vi "Close_Refs.vi"(8 "Error In":errorcluster caption="Entrée d'erreur", 11 "Donnees_Globales_IN":T1) -> (0 "Error Out":errorcluster)   [LabVIEW 2019]
uses:
  Asc_State_Inputs.ctl
  Etat_Asc.ctl
  <vilib>/Utility/error.llb/Error Cluster From Error Code.vi
  <vilib>/rvi/errors/niLvFpgaAdjustHostInterfaceError.vi
  <vilib>/FPGAPlugInAG/Dynamic/niLvFpga_Close_Dynamic.vi
  <vilib>/rvi/interface/nirviReadWriteControl/nirviReadWriteControl.xnode
  <vilib>/rvi/interface/nirviCloseFPGA/nirviCloseFPGA.xnode
  NiFpgaLv.dll
  <vilib>/rvi/interface/Simulation/niFpgaSimulationCallBeginRW.vi
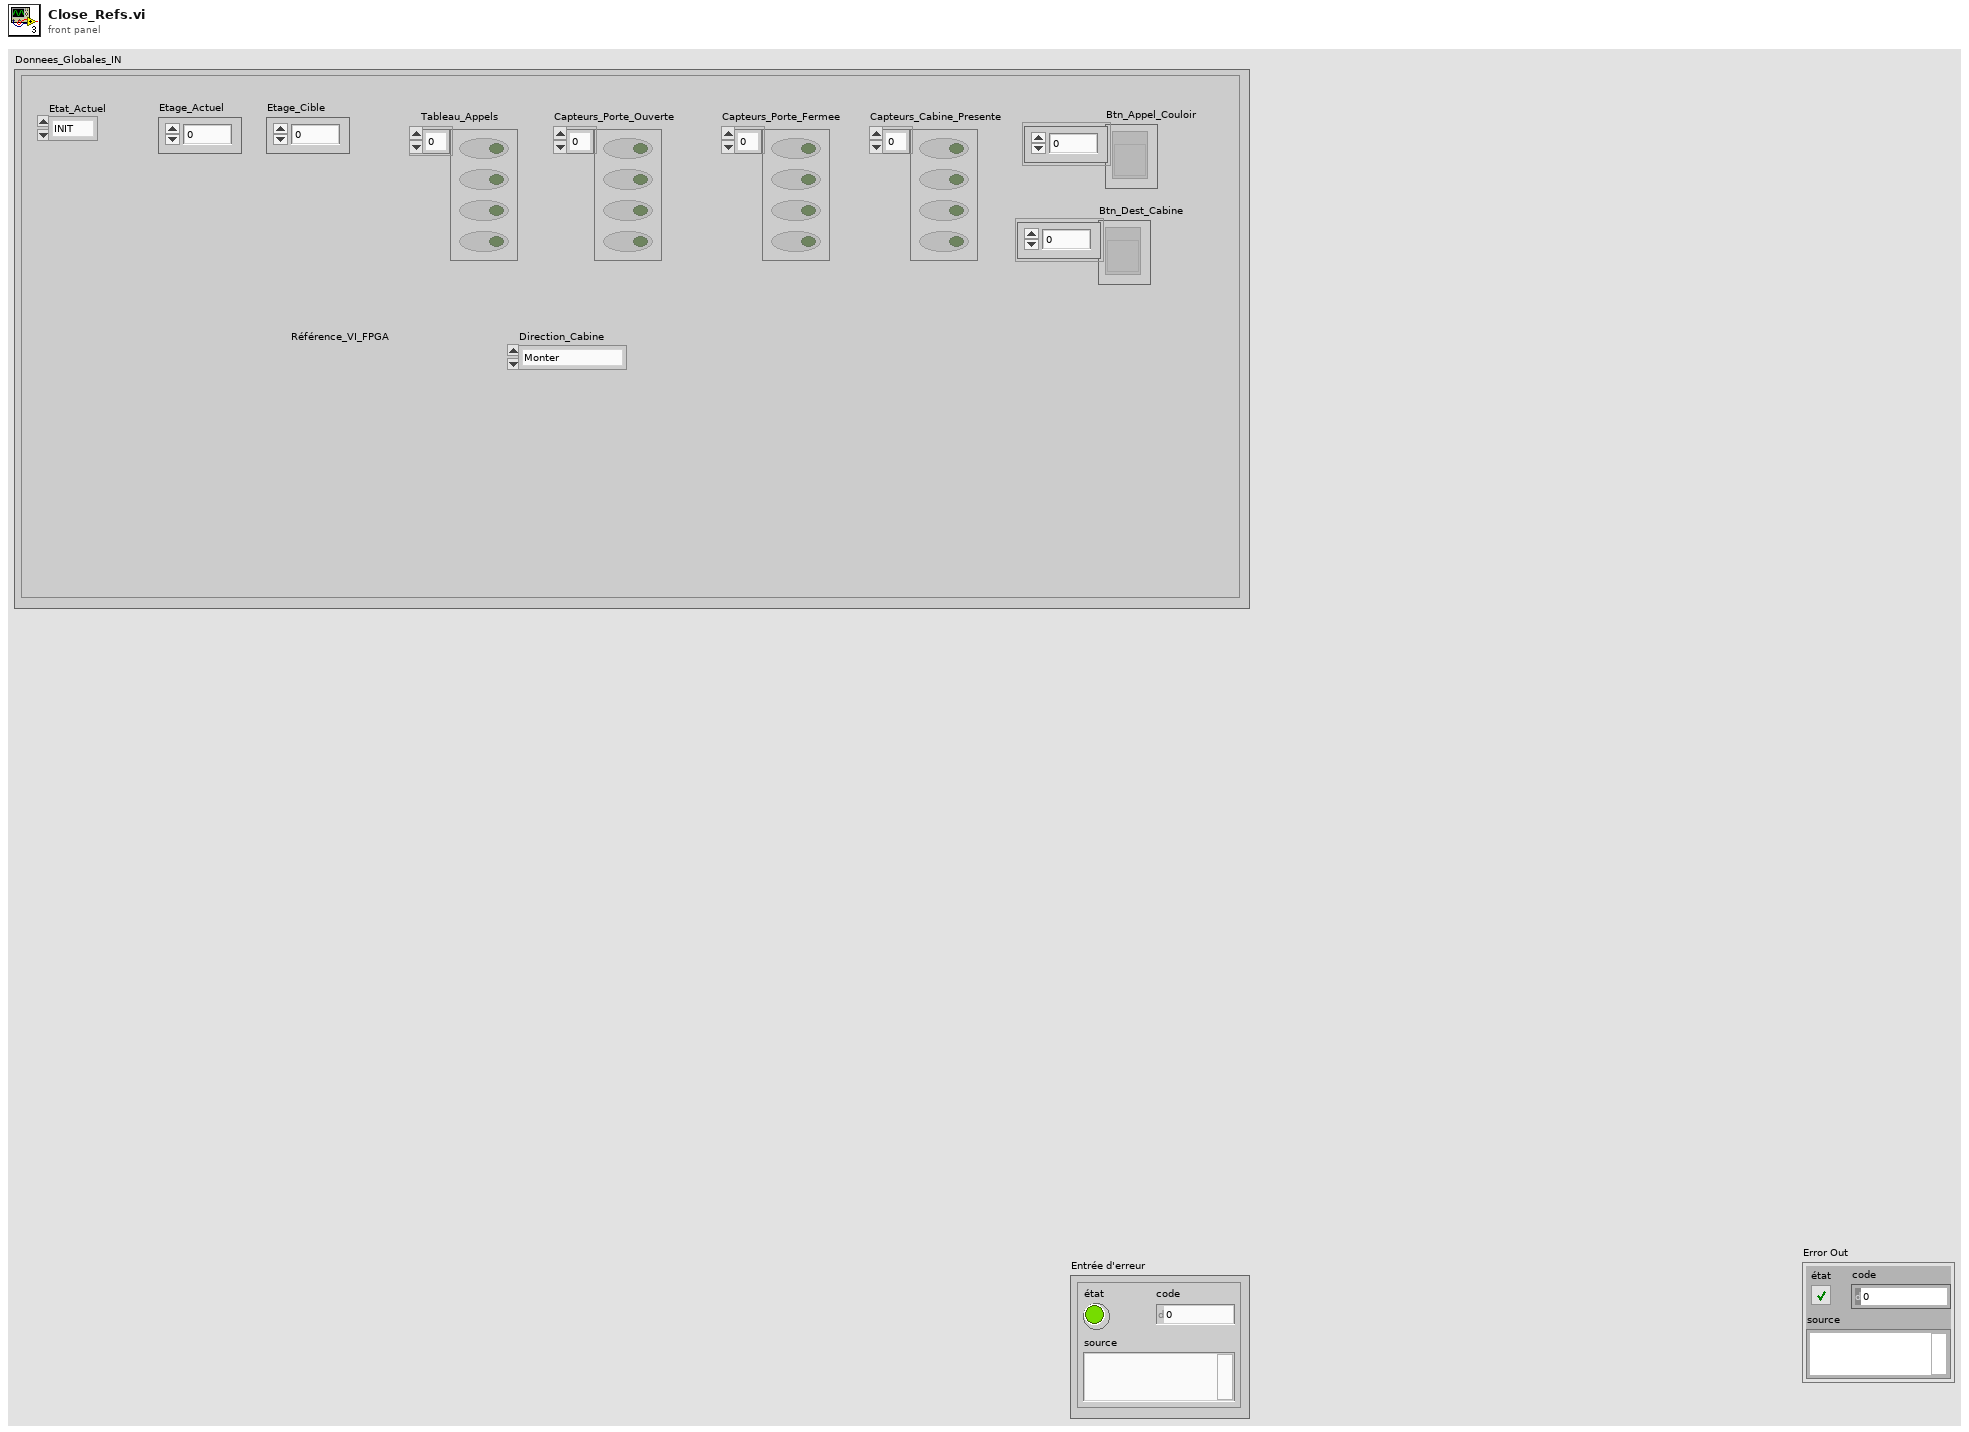
[diagram p1: front panel]
types:
  T1 = typedef "Asc_State_Inputs.ctl" = cluster{"Etage_Actuel":i32, "Etat_Actuel":T2, "Etage_Cible":i32, "Tableau_Appels":bool[], "Capteurs_Porte_Ouverte":bool[], "Capteurs_Porte_Fermee":bool[], "Capteurs_Cabine_Presente":bool[], "Btn_Appel_Couloir":refnum<vi>[], "Btn_Dest_Cabine":refnum<vi>[], "Référence_VI_FPGA":refnum<k20>, "Direction_Cabine":enum16{"Monter", "Descendre", "Arreter"}}
  T2 = typedef "Etat_Asc.ctl" = enum16{"INIT", "REPOS", "DEPLACEMENT", "OUVERTURE_PORTE", "ATTENTE_TEMPO", "FERMETURE_PORTE", "ARRET_URGENCE"}
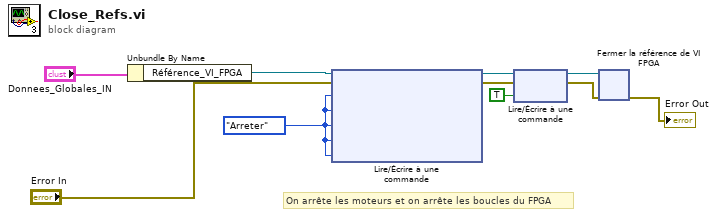
[diagram p0: block diagram]
diagram:
  w7 = enum16{"Monter", "Descendre", "Arreter"}."Arreter" ("CMD_Moteur_Cabine")
  # "On arrête les moteurs et on arrête les boucles du FPGA"
  n1 = Unbundle By Name("Donnees_Globales_IN") -> ("Référence_VI_FPGA"=w8:refnum<k20>)
  n2 = xnode "Lire/Écrire à une commande"("Référence de VI FPGA en entrée"=w8, "entrée d'erreur"="Error In", "CMD_Moteur_Cabine"=w7, "CMD_Moteur_Porte_RDC"=w7, "CMD_Moteur_Porte_1"=w7, "CMD_Moteur_Porte_2"=w7, "CMD_Moteur_Porte_3"=w7) -> ("Référence de VI FPGA en sortie"=w6:refnum<k20>, "sortie d'erreur"=w5:errorcluster)
  n3 = xnode "Lire/Écrire à une commande"("Référence de VI FPGA en entrée"=w6, "entrée d'erreur"=w5, "STOP"=TRUE) -> ("Référence de VI FPGA en sortie"=w2:refnum<k20>, "sortie d'erreur"=w1:errorcluster)
  n4 = xnode "Fermer la référence de VI FPGA"("Référence de VI FPGA en entrée"=w2, "entrée d'erreur"=w1) -> ("sortie d'erreur"=→"Error Out":errorcluster)
